vi "Teleop.vi"(10 "Match Info":T1={"Autonomous Elapsed Seconds"=0.0, "TeleOp Elapsed Seconds"=0.0, "Disabled Elapsed Seconds"=0.0, "Visited Autonomous"=FALSE, "Visited TeleOp"=FALSE, "Visited Disabled"=FALSE, "Autonomous Settings"={"Autonomous Style"=enum."Independent", "VI Refnum"=refnum}}, 11 "Call Context":T2) -> ()   [LabVIEW 2015]
doc: "This VI is called for each TeleOp packet received from the DS where the robot is not disabled. It is often used to read from the joysticks and update I/O or to update setpoints for timed control loops. It should complete and return within 20 milliseconds or it may miss DS packets."
uses:
  <vilib>/Rock Robotics/WPI/DriverStation/WPI_DriverStationDerivedRobotMode.ctl
  <vilib>/Rock Robotics/WPI/DriverStation/WPI_DriverStationMatch Info.ctl
  <userlib>/836-Library/Pneumatics/Support Code/Pneumatics Command.ctl
  <vilib>/Rock Robotics/WPI/Utilities/WPI_GetSetVariantRefNum.vi
  <userlib>/836-Library/Pneumatics/Support Code/Pneumatics Command Set Tele.vi
  Pneumatic Commands.ctl
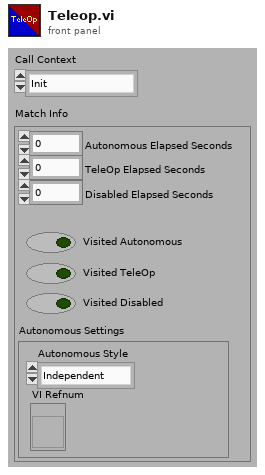
[diagram p1: front panel]
types:
  T1 = typedef "WPI_DriverStationMatch Info.ctl" = cluster{"Autonomous Elapsed Seconds":dbl, "TeleOp Elapsed Seconds":dbl, "Disabled Elapsed Seconds":dbl, "Visited Autonomous":bool, "Visited TeleOp":bool, "Visited Disabled":bool, "Autonomous Settings":cluster{"Autonomous Style":enum16{"Iterative", "Independent"}, "VI Refnum":refnum<vi>}}
  T2 = typedef "WPI_DriverStationDerivedRobotMode.ctl" = enum16{"Init", "Execute", "Stop"}
  T3 = typedef "WPI_JoystickDevRef.ctl" = cluster{"Device":T4}
  T4 = typedef "WPI_JoystickDeviceEnum.ctl" = enum16{"USB 0", "USB 1", "USB 2", "USB 3", "USB 4", "USB 5"}
  T5 = typedef "Pneumatic Commands.ctl" = enum16{"Go Up", "Go Down", "Nothing"}
  T6 = typedef "Pneumatics Command.ctl" = enum16{"Nothing", "Forward", "Reverse", "Toggle"}
  T7 = typedef "WPI_MotorControlDeviceRef.ctl" = cluster{"DeviceStatus":errorcluster, "Type":T8, "PWM":cluster{"PWM Channel":T9, "DeadBand":T10}, "CAN":cluster{"Device Number":u8, "Control Mode":T11, "Semaphore":T12, "Max Vout":dbl, "TalonSRX Control Mode":T13}, "Invert":bool}
  T8 = typedef "WPI_MotorControlType.ctl" = enum16{"PWM", "CAN", "CANTalonSRX"}
  T9 = typedef "FPGA_DIOPWMChannel.ctl" = enum8{"PWM 0", "PWM 1", "PWM 2", "PWM 3", "PWM 4", "PWM 5", "PWM 6", "PWM 7", "PWM 8", "PWM 9", "PWM MXP 0", "PWM MXP 1", "PWM MXP 2", "PWM MXP 3", "PWM MXP 4", "PWM MXP 5", "PWM MXP 6", "PWM MXP 7", "PWM MXP 8", "PWM MXP 9", "Invalid"}
  T10 = typedef "WPI_PWMDeadband.ctl" = cluster{"Name":string, "maxPositivePwm":i32, "minPositivePwm":i32, "centerPwm":i32, "maxNegativePwm":i32, "minNegativePwm":i32, "angularRange":u16}
  T11 = typedef "WPI_CANJaguar_ControlMode.ctl" = enum8{"Percent VBus", "Current", "Speed", "Position", "Voltage"}
  T12 = typedef "Semaphore RefNum" = refnum<k1>
  T13 = typedef "WPI_CANTalonSRX_APIControlMode.ctl" = enum8{"Percent VBus", "Speed", "Position", "Slave", "Unchanged / Invalid", "Voltage Compensation", "Current", "Motion Profile"}
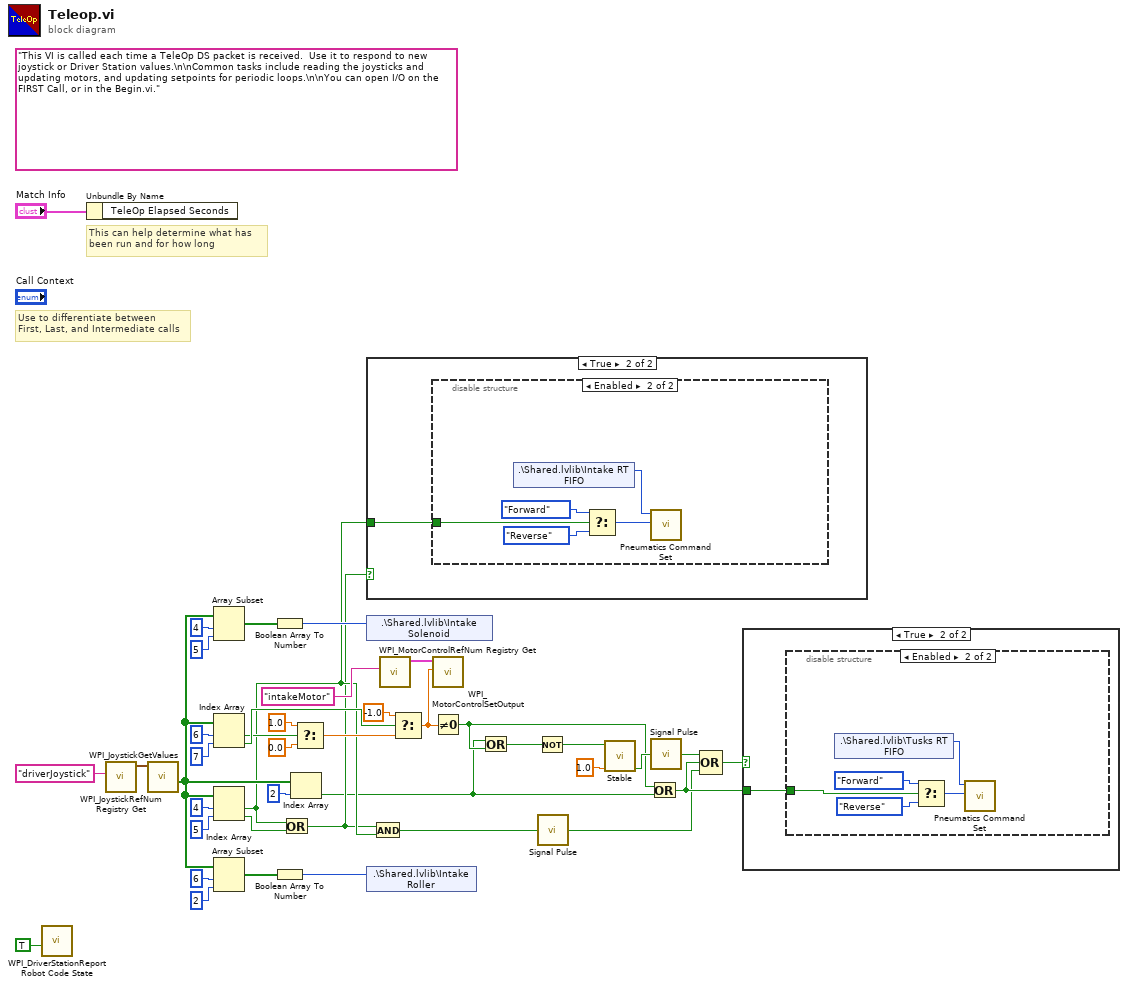
[diagram p0: block diagram]
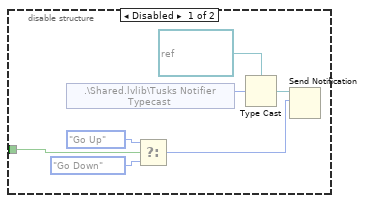
[diagram p3: hidden frame]
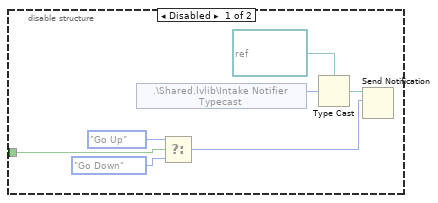
[diagram p5: hidden frame]
diagram:
  (unwired) "This VI is called each time a TeleOp DS packet is received.  Use it to respond to new joystick or Driver Station values.\n\nCommon tasks include reading the joysticks and updating motors, and updating setpoints for periodic loops.\n\nYou can open I/O on the FIRST Call, or in the Begin.vi."
  # "Use to differentiate between\nFirst, Last, and Intermediate calls"
  # "This can help determine what has\nbeen run and for how long"
  n1 = call <vilib>:"WPI_DriverStationReport Robot Code State.vi"("TeleOp"=TRUE ("Autonomous")) -> ()  [unwired: 10 in, 1 out]
  n2 = Unbundle By Name("Match Info") -> ()  [unwired: 1 out]
  n3 = call <vilib>:"WPI_JoystickRefNum Registry Get.vi"("refnum name"="driverJoystick") -> ("JoystickDevRef"=w36:T3)  [unwired: 1 in, 9 out]
  n4 = call <vilib>:"WPI_JoystickGetValues.vi"("JoystickDevRef"=w36) -> ("Buttons"=w16:bool[])  [unwired: 6 in, 4 out]
  n5 = Array Subset(array=w16, index=4, length=5) -> (w21:bool[])
  n6 = Index Array(array=w16, index #1=6 ("index"), index #2=7 ("index")) -> (element #1=w34:bool, element #2=w35:bool)
  n7 = Index Array(array=w16, index #1=4 ("index"), index #2=5 ("index")) -> (element #1=w13:bool, element #2=w37:bool)
  n8 = Array Subset(array=w16, index=6, length=2) -> (w22:bool[])
  n9 = Boolean Array To Number(Boolean array=w21) -> (number=w18:u32)
  n10 = Boolean Array To Number(Boolean array=w22) -> (number=w17:u32)
  n11 = Or(x=w13, y=w37) -> (x .or. y?=w12:bool)
  n12 = Index Array(array=w16, index=2) -> (element=w1:bool)
  n13 = Select(t=1.0, s=w34, f=0.0) -> (s? t:f=w32:dbl)
  n14 = case shown="True" w12 {
    tunnel: w13 -> [_ w42]
    frame False {
    }
    frame True {
      n15 = disable-structure shown="Enabled" {
        disable-tunnel: w42 -> [w46 w52]
        frame Disabled {
          w45 = refnum<notifier> refnum items=["Go Up", "Go Down", "Nothing"] ("notifier out")
          n16 = shared-variable ".\\Shared.lvlib\\Intake Notifier Typecast"() -> (w44:u32)  [unwired: 1 in, 1 out]
          n17 = Select(t=Pneumatic_Commands."Go Up", s=w46, f=Pneumatic_Commands."Go Down") -> (s? t:f=w47:T5)
          n18 = Type Cast(type=w45, x=w44) -> (*(type *) &x=w43:refnum<notifier>)
          n19 = Send Notification(notification=w47, notifier=w43) -> ()  [unwired: 1 in, 2 out]
        }
        frame Enabled {
          n20 = shared-variable ".\\Shared.lvlib\\Intake RT FIFO"() -> (w50:u64)  [unwired: 1 in, 1 out]
          n21 = Select(t=Pneumatics_Command."Forward" ("Solenoid Command"), s=w52, f=Pneumatics_Command."Reverse" ("Solenoid Command")) -> (s? t:f=w51:T6)
          n22 = call-poly <userlib>:"Pneumatics Command Set.vi"("Solenoid Command"=w51, "RT FIFO"=w50) -> ()  [unwired: 9 in, 1 out]
        }
      }
    }
  }
  n23 = shared-variable ".\\Shared.lvlib\\Intake Solenoid"(w18) -> ()  [unwired: 1 in, 1 out]
  n24 = shared-variable ".\\Shared.lvlib\\Intake Roller"(w17) -> ()  [unwired: 1 in, 1 out]
  n25 = And(x=w12, y=w13) -> (x .and. y?=w11:bool)
  n26 = call <vilib>:"WPI_MotorControlRefNum Registry Get.vi"("refnum name"="intakeMotor") -> ("MotorControlDevRef"=w26:T7)  [unwired: 9 in, 1 out]
  n27 = Select(t=-1.0 ("f"), s=w35, f=w32) -> (s? t:f=w15:dbl)
  n28 = call <vilib>:"WPI_MotorControlSetOutput.vi"("Output"=w15, "MotorControlDevRef"=w26) -> ()  [unwired: 7 in, 3 out]
  n29 = Not Equal To 0?(x=w15) -> (x != 0?=w4:bool)
  n30 = Or(x=w1, y=w4) -> (x .or. y?=w3:bool)
  n31 = Not(x=w3) -> (.not. x?=w5:bool)
  n32 = call <userlib>:"Signal Pulse.vi"("Input"=w11) -> ("Output"=w2:bool)
  n33 = call <userlib>:"Stable.vi"("Eval Period (sec)"=1.0, "Signal Input"=w5) -> ("Stable"=w8:bool)  [unwired: 9 in]
  n34 = Or(x=w4, y=w1) -> (x .or. y?=w9:bool)
  n35 = call <userlib>:"Signal Pulse.vi"("Input"=w8) -> ("Output"=w6:bool)
  n36 = Compound Arithmetic op=OR(w6, w9, w2) -> (w10:bool)
  n37 = case shown="True" w10 {
    tunnel: w9 -> [_ w55]
    frame False {
    }
    frame True {
      n38 = disable-structure shown="Enabled" {
        disable-tunnel: w55 -> [w56 w64]
        frame Disabled {
          w59 = refnum<notifier> refnum items=["Go Up", "Go Down", "Nothing"] ("notifier out")
          n39 = shared-variable ".\\Shared.lvlib\\Tusks Notifier Typecast"() -> (w57:u32)  [unwired: 1 in, 1 out]
          n40 = Select(t=Pneumatic_Commands."Go Up", s=w56, f=Pneumatic_Commands."Go Down") -> (s? t:f=w60:T5)
          n41 = Type Cast(type=w59, x=w57) -> (*(type *) &x=w58:refnum<notifier>)
          n42 = Send Notification(notification=w60, notifier=w58) -> ()  [unwired: 1 in, 2 out]
        }
        frame Enabled {
          n43 = shared-variable ".\\Shared.lvlib\\Tusks RT FIFO"() -> (w63:u64)  [unwired: 1 in, 1 out]
          n44 = Select(t=Pneumatics_Command."Forward" ("Solenoid Command"), s=w64, f=Pneumatics_Command."Reverse" ("Solenoid Command")) -> (s? t:f=w67:T6)
          n45 = call-poly <userlib>:"Pneumatics Command Set.vi"("Solenoid Command"=w67, "RT FIFO"=w63) -> ()  [unwired: 9 in, 1 out]
        }
      }
    }
  }
